vi "ConvertGoop3ToGoop4_Log.vi"(7 "Action(Enter)":T1, 8 "error in (no error)":errorcluster, 11 "Object":variant) -> (0 "error out":errorcluster, 1 "State":string, 3 "LastItem":string)   [LabVIEW 2020]
uses:
  ConvertGoop3ToGoop4_LogType.ctl
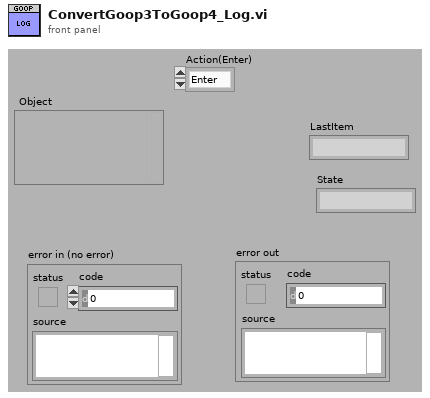
[diagram p1: front panel]
types:
  T1 = typedef "ConvertGoop3ToGoop4_LogType.ctl" = enum16{"Enter", "Read"}
  T2 = enum16{"open", "replace", "create", "open or create", "replace or create", "replace or create with confirmation"}
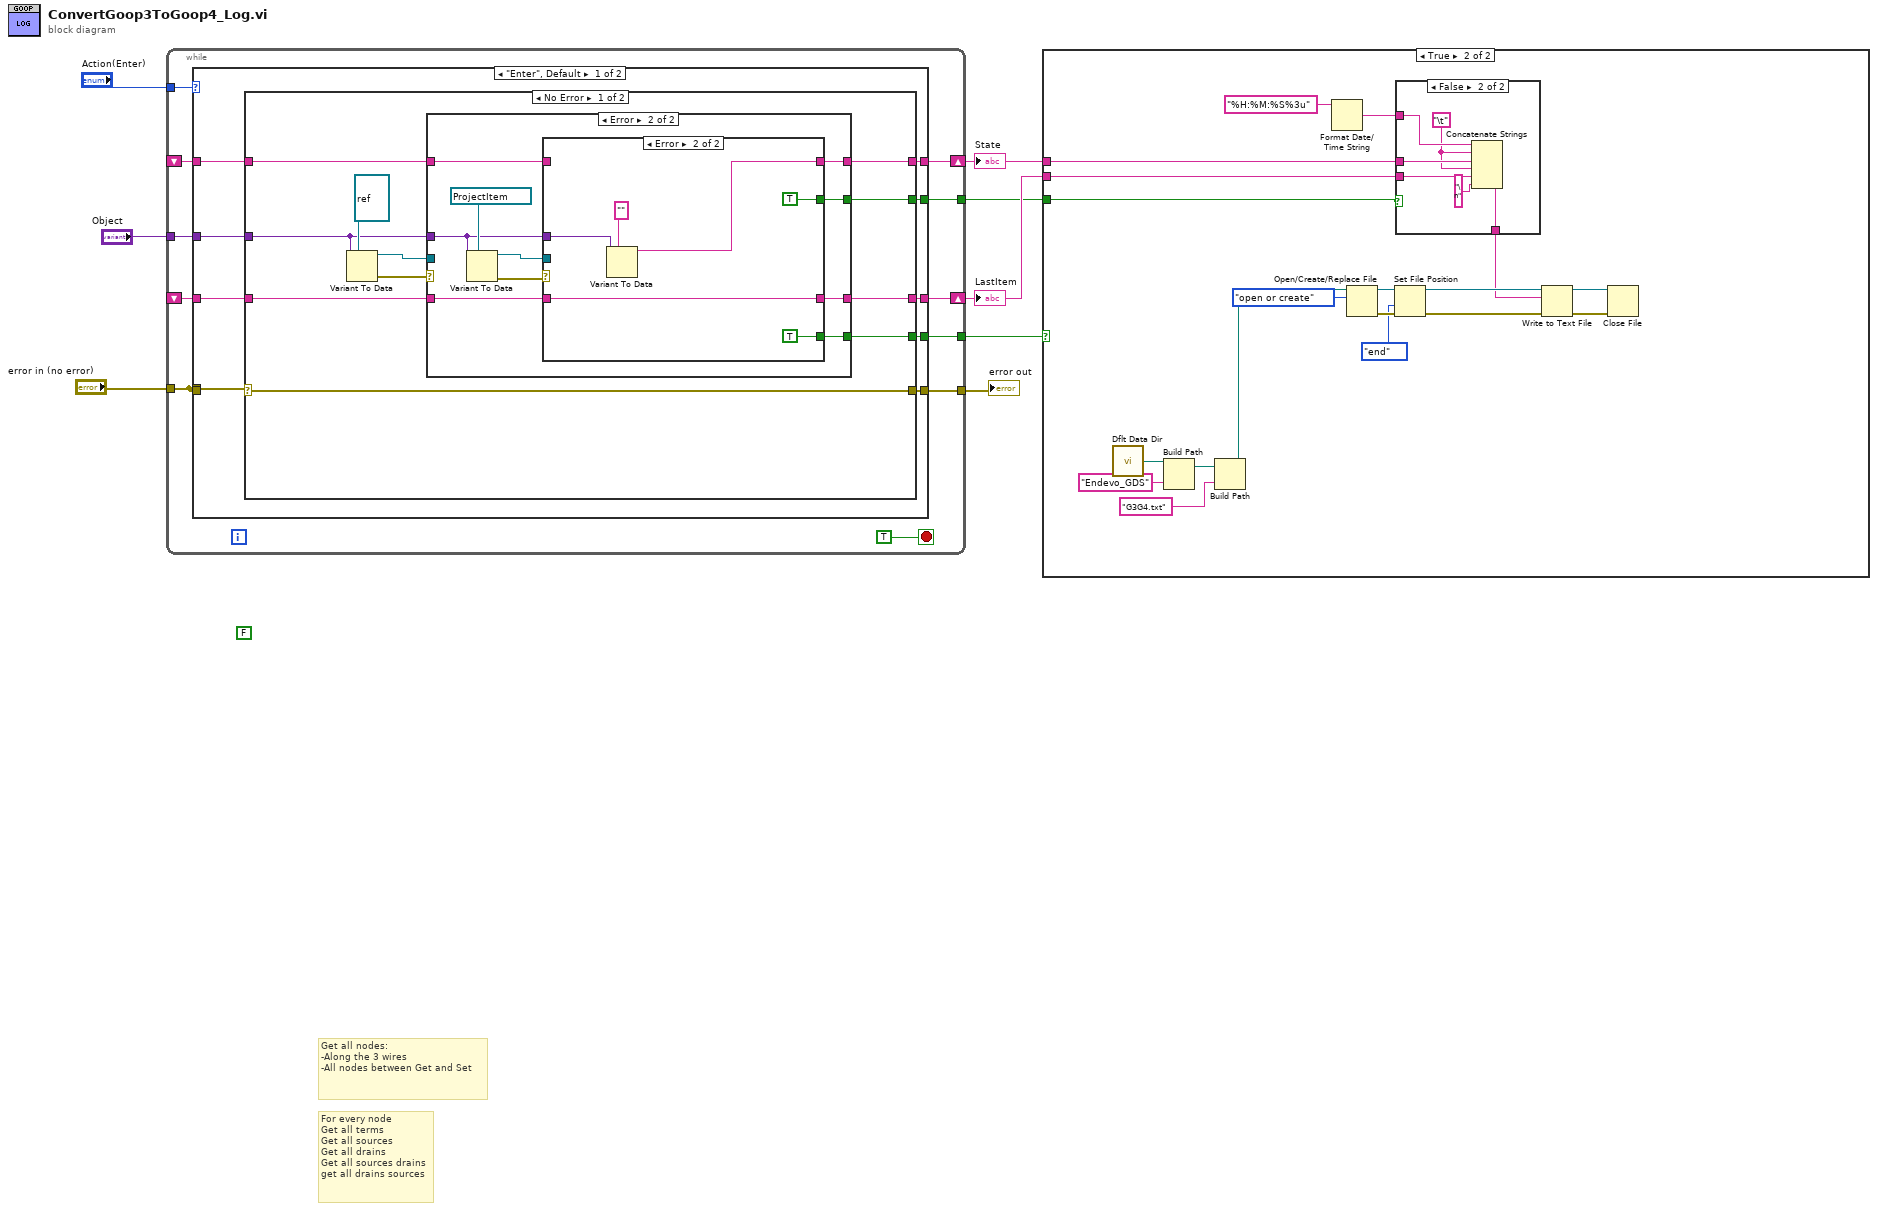
[diagram p0: block diagram]
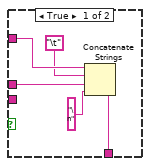
[diagram p3: hidden frame]
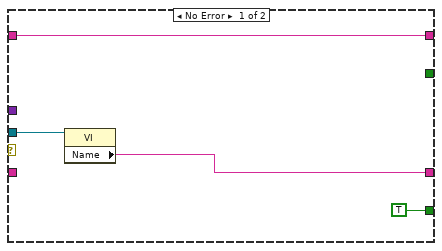
[diagram p4: hidden frame]
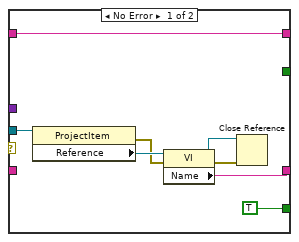
[diagram p5: hidden frame]
diagram:
  (unwired) FALSE ("Block Diagram Window:Open")
  # "For every node\nGet all terms\nGet all sources\nGet all drains\nGet all sources drains\nget all drains sources"
  # "Get all nodes:\n-Along the 3 wires\n-All nodes between Get and Set"
  n1 = while {
    tunnel: "Object" -> [w19]
    tunnel: "error in (no error)" -> [w13]
    tunnel: [w18] -> w6
    tunnel: "Action(Enter)" -> [w17]
    shift-right: [w15] -> w3
    shift-left: _ -> [w14]
    shift-right: [w12] -> w1
    shift-left: _ -> [w11]
    tunnel: [w10] -> w4
    tunnel: [w9] -> w2
    stop <- TRUE stop-if-true
    n2 = case shown="\"Enter\", Default" w17 {
      tunnel: w19 -> [w28 _]
      tunnel: w13 -> [w27 _]
      tunnel: [w26 w72] -> w18
      tunnel: [w25 w73] -> w15
      tunnel: w14 -> [w24 w73]
      tunnel: w13 -> [_ w72]
      tunnel: [w23 w71] -> w12
      tunnel: w11 -> [w22 w71]
      tunnel: [w21 _] -> w10
      tunnel: [w20 _] -> w9
      frame "Enter", Default {
        n3 = case shown="No Error" w27 {
          selector: w27 -> [w33 w70]
          tunnel: w28 -> [w38 _]
          tunnel: [w33 w70] -> w26
          tunnel: [w35 w69] -> w25
          tunnel: w24 -> [w34 w69]
          tunnel: [w32 w68] -> w23
          tunnel: w22 -> [w31 w68]
          tunnel: [w30 _] -> w21
          tunnel: [w29 _] -> w20
          frame No Error {
            n4 = Variant To Data(type=refnum<vi> refnum ("reference"), Variant=w38) -> (data=w36:refnum<vi>, error out=w37:errorcluster)  [unwired: 1 in]
            n5 = case shown="Error" w37 {
              tunnel: w38 -> [_ w48]
              tunnel: w36 -> [w43 _]
              tunnel: [w42 w50] -> w35
              tunnel: w34 -> [_ w49]
              tunnel: [w41 w47] -> w32
              tunnel: w31 -> [w41 w46]
              tunnel: [TRUE w45] -> w30
              tunnel: [_ w44] -> w29
              frame No Error {
                n6 = property class="VI"(reference=w43) -> ("Name"=w42:string)  [unwired: 1 in, 2 out]
              }
              frame Error {
                n7 = Variant To Data(type=refnum<vi> refnum ("WhileLoop"), Variant=w48) -> (data=w51:refnum<vi>, error out=w52:errorcluster)  [unwired: 1 in]
                n8 = case shown="Error" w52 {
                  tunnel: w51 -> [w61 _]
                  tunnel: [w59 w67] -> w50
                  tunnel: w49 -> [_ w67]
                  tunnel: w48 -> [_ w66]
                  tunnel: [w55 w64] -> w47
                  tunnel: w46 -> [w55 _]
                  tunnel: [TRUE TRUE] -> w45
                  tunnel: [_ TRUE] -> w44
                  frame No Error {
                    n9 = property class="ProjectItem"(reference=w61) -> (error out=w57:errorcluster, "Reference"=w60:refnum<vi>)  [unwired: 1 in, 1 out]
                    n10 = property class="VI"(reference=w60, error in=w57) -> (reference out=w56:refnum<vi>, error out=w58:errorcluster, "Name"=w59:string)
                    n11 = Close Reference(reference=w56, error in (no error)=w58) -> ()  [unwired: 1 out]
                  }
                  frame Error {
                    n12 = Variant To Data(type="", Variant=w66) -> (data=w64:string)  [unwired: 1 in, 1 out]
                  }
                }
              }
            }
          }
          frame Error {
          }
        }
      }
      frame "Read" {
      }
    }
  }
  "error out" <- w6
  "LastItem" <- w3
  "State" <- w1
  n13 = case shown="True" w4 {
    tunnel: w1 -> [_ w84]
    tunnel: w3 -> [_ w83]
    tunnel: w2 -> [_ w79]
    frame False {
    }
    frame True {
      n14 = call <vilib>:"Dflt Data Dir.vi"() -> ("App:Default Data Directory"=w78:path)
      n15 = Build Path(base path=w78, name or relative path="Endevo_GDS") -> (appended path=w76:path)
      n16 = Build Path(base path=w76, name or relative path="G3G4.txt") -> (appended path=w74:path)
      n17 = Format Date/Time String(time format string (%c)="%H:%M:%S%3u") -> (date/time string=w85:string)  [unwired: 2 in]
      n18 = Open/Create/Replace File(file path (use dialog)=w74, operation (0:open)=T2."open or create") -> (refnum out=w90:refnum<file>, error out=w91:errorcluster)  [unwired: 4 in, 1 out]
      n19 = Set File Position(refnum=w90, from (0:start)=enum16{"start", "end", "current"}."end", error in=w91) -> (refnum out=w88:refnum<file>, error out=w87:errorcluster)  [unwired: 1 in]
      n20 = case shown="False" w79 {
        tunnel: w85 -> [w97 w103]
        tunnel: w84 -> [w96 w102]
        tunnel: w83 -> [_ w100]
        tunnel: [w93 w98] -> w82
        frame True {
          n21 = Concatenate Strings(w97, "\t", w96, "\n" ("string")) -> (w93:string)
        }
        frame False {
          w101 = "\t"
          n22 = Concatenate Strings(w103, w101, w102, w101, w100, "\n" ("string")) -> (w98:string)
        }
      }
      n23 = Write to Text File(file (use dialog)=w88, text=w82, error in=w87) -> (refnum out=w81:refnum<file>, error out=w80:errorcluster)  [unwired: 1 in, 1 out]
      n24 = Close File(refnum=w81, error in=w80) -> ()  [unwired: 2 out]
    }
  }
